vi "RichToFlatnixnet_grpc_BlinkRequest.vi"(5 "OutputClusterType":T1, 11 "InputCluster":T4) -> (3 "OutputCluster":T1)   [LabVIEW 2025, in "grpc-xnet_client.lvlib"]
uses:
  grpc-xnet_client.lvlib
  nixnet_grpc_BlinkRequest.ctl
  nixnet_grpc_BlinkRequest_modifier_enum/nixnet_grpc_BlinkRequest_modifier_enum.lvclass
  nidevice_grpc_Session.ctl
  nixnet_grpc_BlinkRequest_Flat.ctl
  nidevice_grpc_Session_Flat.ctl
  nixnet_grpc_BlinkMode.ctl
  nixnet_grpc_BlinkRequest_modifier_enum/nixnet_grpc_BlinkRequest_modifier_enum.lvclass/nixnet_grpc_BlinkRequest_modifier_enum.ctl
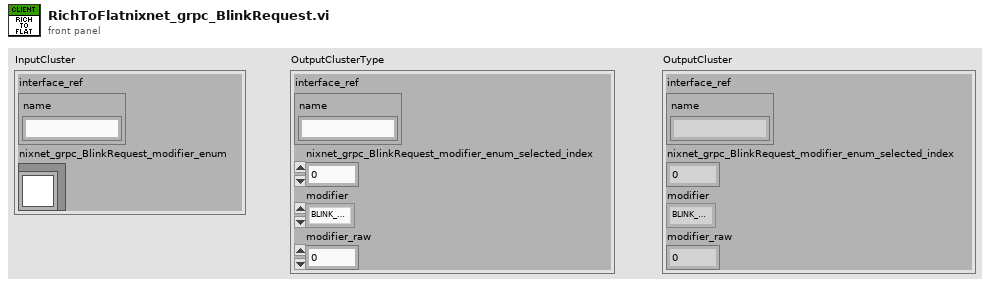
[diagram p1: front panel]
types:
  T1 = typedef "grpc-xnet_client.lvlib/nixnet_grpc_BlinkRequest_Flat.ctl" = cluster{"interface_ref":T2, "nixnet_grpc_BlinkRequest_modifier_enum_selected_index":i32, "modifier":T3, "modifier_raw":u32}
  T2 = typedef "grpc-xnet_client.lvlib/nidevice_grpc_Session_Flat.ctl" = cluster{"name":string}
  T3 = typedef "grpc-xnet_client.lvlib/nixnet_grpc_BlinkMode.ctl" = enum32{"BLINK_MODE_DISABLE", "BLINK_MODE_ENABLE"}
  T4 = typedef "grpc-xnet_client.lvlib/nixnet_grpc_BlinkRequest.ctl" = cluster{"interface_ref":T5, "nixnet_grpc_BlinkRequest_modifier_enum":refnum<class "nixnet_grpc_BlinkRequest_modifier_enum.lvclass">}
  T5 = typedef "grpc-xnet_client.lvlib/nidevice_grpc_Session.ctl" = cluster{"name":string}
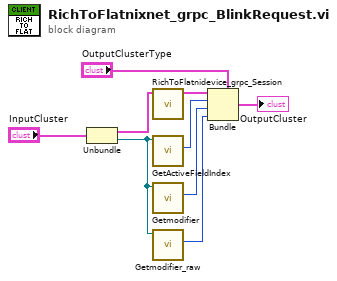
[diagram p0: block diagram]
diagram:
  n1 = Unbundle "Unbundle"("InputCluster") -> ("interface_ref"=w6:T5, "nixnet_grpc_BlinkRequest_modifier_enum"=w4:refnum<class "nixnet_grpc_BlinkRequest_modifier_enum.lvclass">)
  n2 = call "RichToFlatnidevice_grpc_Session.vi"("InputCluster"=w6) -> ("OutputCluster"=w5:T2)  [unwired: 10 in]
  n3 = call "GetActiveFieldIndex.vi"("OneOfTemplate in"=w4) -> ("Active Field Index"=w3:i32)  [unwired: 8 in, 2 out]
  n4 = call "Getmodifier.vi"("OneOfTemplate in"=w4) -> ("Get_Val"=w2:T3)  [unwired: 8 in, 2 out]
  n5 = call "Getmodifier_raw.vi"("OneOfTemplate in"=w4) -> ("Get_Val"=w1:u32)  [unwired: 8 in, 2 out]
  n6 = Bundle "Bundle"(cluster="OutputClusterType", "interface_ref"=w5, "nixnet_grpc_BlinkRequest_modifier_enum_selected_index"=w3, "modifier"=w2, "modifier_raw"=w1) -> (→"OutputCluster":T1)
